vi "AutoDrive.vi"(10 "Distance":dbl, 11 "Angle":dbl) -> ()   [LabVIEW 2017]
panel:
  in  "Complete":bool
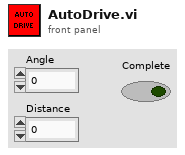
[diagram p1: front panel]
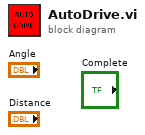
[diagram p0: block diagram]
diagram:
